vi "write IO variable I16.vi"(8 "error in (no error)":errorcluster, 9 "Command/Value":i16, 10 "Index":i32, 11 "IO Variable Array In":refnum<k21>[](array[refnum])) -> (0 "error out":errorcluster, 3 "IO Variable Array Out":refnum<k21>[](array[refnum]))   [LabVIEW 2016, in "Scan Engine Custom Device.lvlib" / "DS402.lvlib"]
uses:
  DS402.lvlib
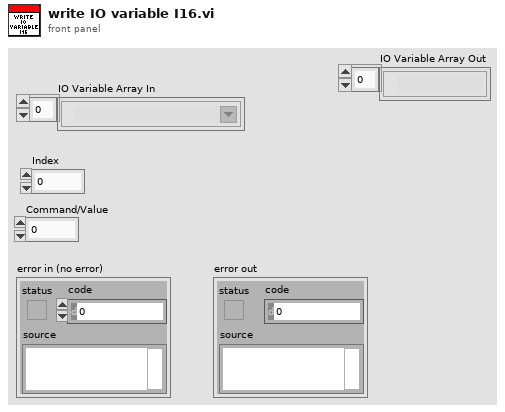
[diagram p1: front panel]
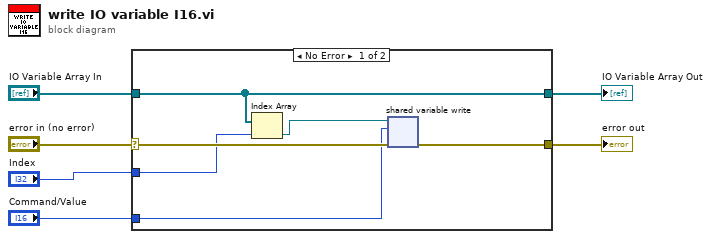
[diagram p0: block diagram]
diagram:
  n1 = case shown="No Error" "error in (no error)" {
    selector: "error in (no error)" -> [w10 w14]
    tunnel: [w12 w14] -> w6
    tunnel: "IO Variable Array In" -> [w8 w13]
    tunnel: "Index" -> [w9 _]
    tunnel: [w8 w13] -> w2
    tunnel: "Command/Value" -> [w7 _]
    frame No Error {
      n2 = Index Array(array=w8, index=w9) -> (element=w11:refnum<k21>)
      n3 = shared-variable-write(w11, w10, w7) -> (w12:errorcluster)  [unwired: 1 out]
    }
    frame Error {
    }
  }
  "error out" <- w6
  "IO Variable Array Out" <- w2
